vi "Destroy User Event.vi"(8 "Error In":errorcluster, 11 "User Event Reference":T1) -> (0 "Error Out":errorcluster)   [LabVIEW 2023, in "QSM - Alarms.lvlib"]
doc: "This VI destroys the user event for the Queued Message Handler template."
uses:
  QSM - Alarms.lvlib
  Controls/User Event Type.ctl
  Controls/User Event Reference.ctl
  Controls/Event Handler Message.ctl
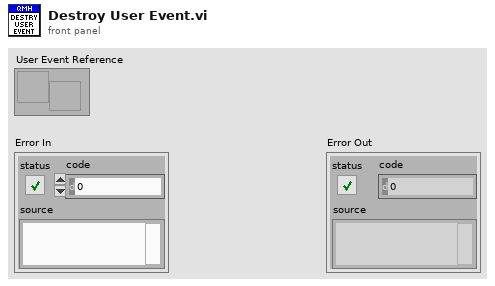
[diagram p1: front panel]
types:
  T1 = typedef "QSM - Alarms.lvlib/User Event Reference.ctl" = refnum<user-event>
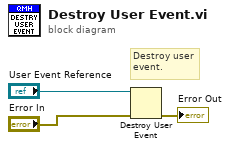
[diagram p0: block diagram]
diagram:
  # "Destroy user\nevent."
  n1 = Destroy User Event(user event="User Event Reference", error in="Error In") -> (error out=→"Error Out":errorcluster)
